vi "UDP Communication.vi"(8 "error in":errorcluster) -> ()   [LabVIEW 2011]
doc: "This VI runs in parallel to other tasks. It can contain as many user-defined periodic loops as you need. These can carry out PID or other sorts of timed response."
uses:
  UDP Dashboard Packet TypeDef.ctl
  Robot Global Data.vi
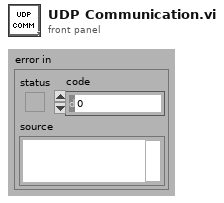
[diagram p1: front panel]
types:
  T1 = typedef "UDP Dashboard Packet TypeDef.ctl" = cluster{"Distance":dbl}
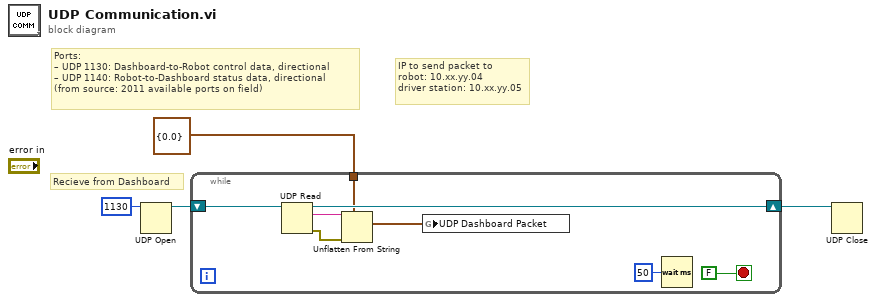
[diagram p0: block diagram]
diagram:
  # "IP to send packet to \nrobot: 10.xx.yy.04\ndriver station: 10.xx.yy.05"
  # "Recieve from Dashboard"
  # "Ports:\n– UDP 1130: Dashboard-to-Robot control data, directional\n– UDP 1140: Robot-to-Dashboard status data, directional\n(from source: 2011 available ports on field)"
  n1 = UDP Open(11:u16 1130 ("port")) -> (port=w3:refnum<k16>)  [unwired: 4 in, 2 out]
  n2 = while {
    shift-right: [w11] -> w2
    shift-left: w3 -> [w10]
    tunnel: T1 {"Distance"=0.0} ("UDP Dashboard Packet") -> [w7]
    stop <- FALSE stop-if-true
    n3 = UDP Read(connection ID=w10) -> (data out=w8:string, error out=w9:errorcluster, 3:w11:refnum<k16>)  [unwired: 3 in, 2 out]
    n4 = Unflatten From String(type=w7, binary string=w8, error in (no error)=w9) -> (value=w6:T1)  [unwired: 2 in, 2 out]
    n5 = global write "Robot Global Data.vi" "UDP Dashboard Packet"(w6) -> ()
    n6 = Wait (ms)(milliseconds to wait=u32 50) -> ()  [unwired: 1 out]
  }
  n7 = UDP Close(connection ID=w2) -> ()  [unwired: 1 in, 2 out]
